vi "BMcalculate_v2_2.vi"() -> ()   [LabVIEW 2016]
uses:
  <vilib>/Analysis/coordinate.llb/2D Cartesian Coordinate Rotation (Array).vi
  <vilib>/Analysis/baseanly.llb/Mean (DBL).vi
  <vilib>/Utility/file.llb/Read From Spreadsheet File (string).vi
  <vilib>/Utility/file.llb/Write To Spreadsheet File (DBL).vi
  <vilib>/Analysis/NI_AALBase.lvlib
  <vilib>/Analysis/NI_AALPro.lvlib
panel:
  out "yBM (delete x/y,R2)":dbl[](array[numeric])
  out "xBM (delete x/y,R2)":dbl[](array[numeric])
  out "aoi count (delete x/y)":dbl[](array[numeric])
  out "y position (delete x/y)":dbl[][](array[numeric])
  out "yBM (delete x/y)":dbl[](array[numeric])
  out "xBM (delete x/y)":dbl[](array[numeric])
  out "x position (delete x/y)":dbl[][](array[numeric])
  out "aoi count":dbl[](array[numeric])
  out "aoi count repeat":dbl[](array[numeric])
  out "Tandem Yi position":dbl[](array[numeric])
  out "Tandem Xi position":dbl[](array[numeric])
  out "Time trace no hightlight":T1(graph)
  out "frame":i32
  out "BM":dbl[](array[numeric])
  out "sec":dbl[](array[numeric])
  out "y position (pixel) per aoi":dbl[](array[numeric])
  out "x position (pixel) per aoi":dbl[](array[numeric])
  out "final good yBM":dbl[](array[numeric])
  out "final good xBM":dbl[](array[numeric])
  out "final good aois (string)":string[](array[string])
  out "final good aoi (string)":string
  out "final good aois":dbl[](array[numeric])
  out "# of AOIs":dbl
  out "path out":path
  in  "(T=X , F=Y)":bool=TRUE
  in  "Filter window size":i32=100
  out "XYplot":path
  out "TimeTrace":path
  in  "Save Time-trace":bool
  in  "nm/pixel":dbl=72.5 format="%#_13g"
  in  "Folder path":path
  in  "?":bool
  in  "to":dbl=1.15 format="%#_13g"
  in  "x/y for all":dbl=0.85 format="%#_13g"
  out "filename":string
  in  "Filter mode":T2(ring)=enum."Median_slide window"
  in  "Save to vertical data ?":bool
  in  "?":enum32{"slide by slide", "delay"}(tab)=enum."delay"
  in  "?":bool
  in  "seconds to wait":u32
  in  "?":dbl=7.963 format="%#_13g"
  in  "?":dbl=48.61 format="%#_13g"
  in  "Save BM":bool
  in  "?":bool=TRUE
  in  "Save X-Y plot":bool
  in  "less than":dbl=0.2 format="%#_13g"
  in  "?":bool
  in  "?":bool
  in  "?":bool=TRUE
  out "# of frames":dbl
  in  "?":T3(tab)
  out "Filenames":string[](array[string])
  out "useful AOIs":i32[](array[numeric])
  out "# of AOI":i32[](array[numeric])
  out "% of useful AOIs":dbl
  out "tt # of AOIs":i32
  out "# of Frames":dbl[](array[numeric])
  out "tt # 0f useful AOIs":i32
  out "?":T4(graph)
  out "# of useful (each file)":i32
  out "X-Y plot":cluster{dbl[], dbl[]}(graph)
  out "Xstd":dbl
  out "ystd":dbl[](array[numeric])
  out "X":dbl format="%0.2f"
  out "Y":dbl format="%0.2f"
  out "?":T4(graph)
  out "tt # of useful AOIs":i32
  out "xstd":dbl[](array[numeric])
  out "all y position (pixel)":dbl[][](array[numeric])
  out "all x position (pixel)":dbl[][](array[numeric])
  out "Useful aoi number":string[][](array[string])
  in  "Tab Control":enum32{"Time trace"}(tab)
  out "Time trace":T1(graph)
  in  "Highlight":dbl=30.0
  in  "∮":dbl=30.0
  out "aoi":string
  in  "stop frame1":dbl
  in  "start frame1":dbl
  in  "start frame3":dbl
  in  "stop frame2":dbl
  in  "stop frame3":dbl
  in  "start frame2":dbl
  # "Critiria"
  # "∮"
  # "nm"
  # "for ssDNA strande exchange \n                    23.776∮6.613 nm"
  # "for D-loop  (90+4)\n                    48.61∮7.963 nm"
  # "for D-loop  (150+4)\n                    49.57∮8.56 nm"
  # "nm"
  # "Buffer wash"
  # "to"
  # "to"
  # "to"
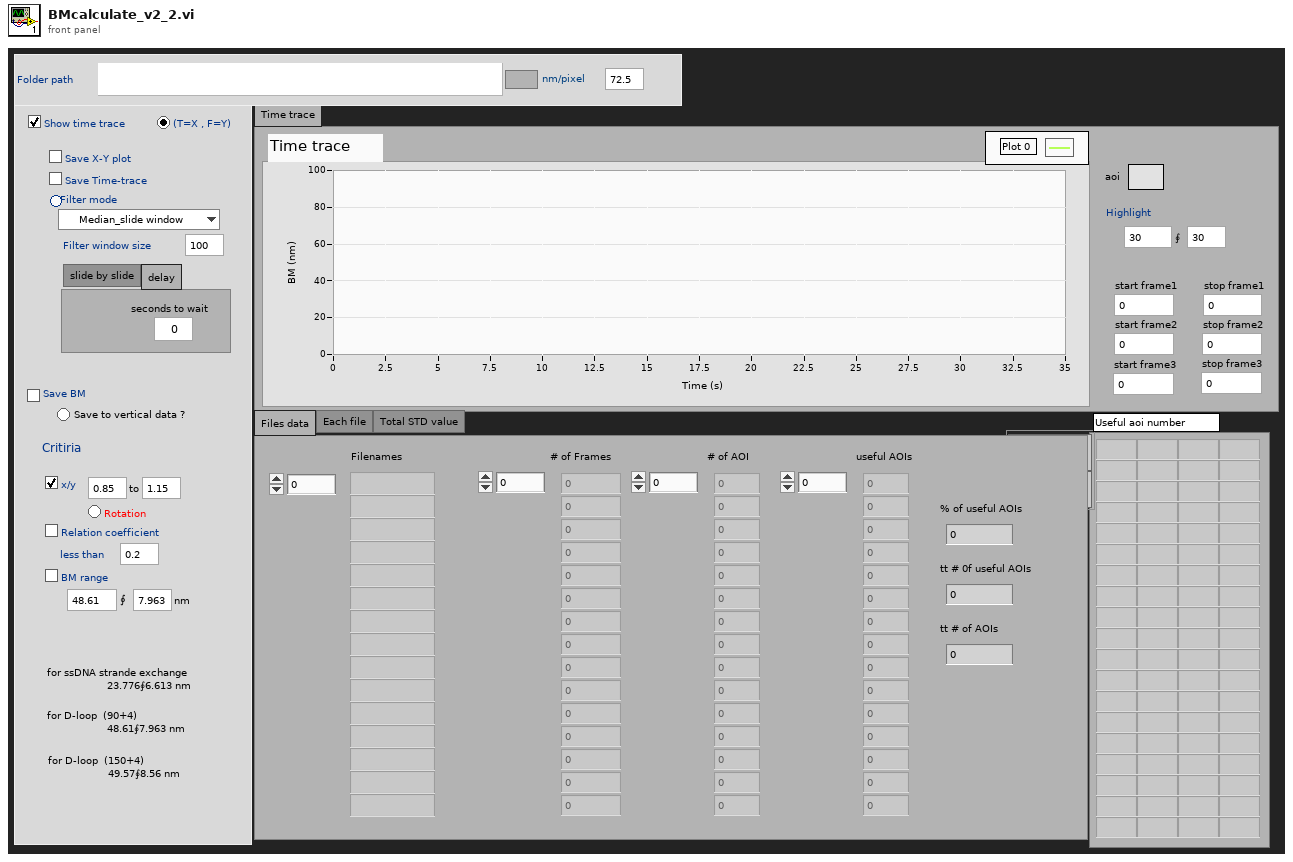
[diagram p1: front panel]
types:
  T1 = cluster{"Filtered X":dbl[], "Filtered X":dbl[]}[]
  T2 = enum16{"Median_fix window", "Average_fix window", "Median_slide window", "Average_slide window"}
  T3 = enum32{"Files data", "Each file", "Total STD value"}
  T4 = cluster{"X Values":dbl[], "Histogram: h(x)":i32[]}
  T5 = cluster{"y position (pixel) per aoi":dbl[], "x position (pixel) per aoi":dbl[]}
  T6 = cluster{"x position (pixel) per aoi":dbl[], "y position (pixel) per aoi":dbl[]}
  T7 = typedef "imagedata.ctl" = cluster{"image type":i32, "image depth":i32, "image":u8[], "mask":u8[], "colors":u32[], "Rectangle":cluster{"left":i16, "top":i16, "right":i16, "bottom":i16}}
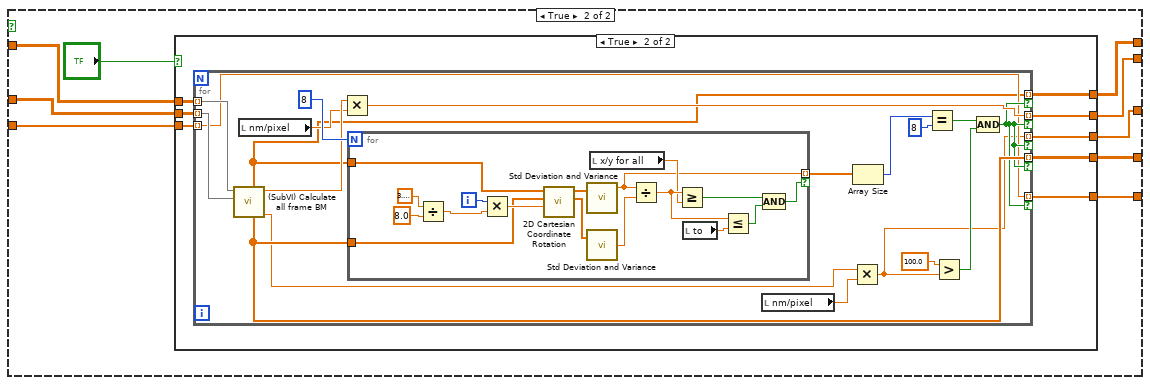
[diagram p3: hidden frame]
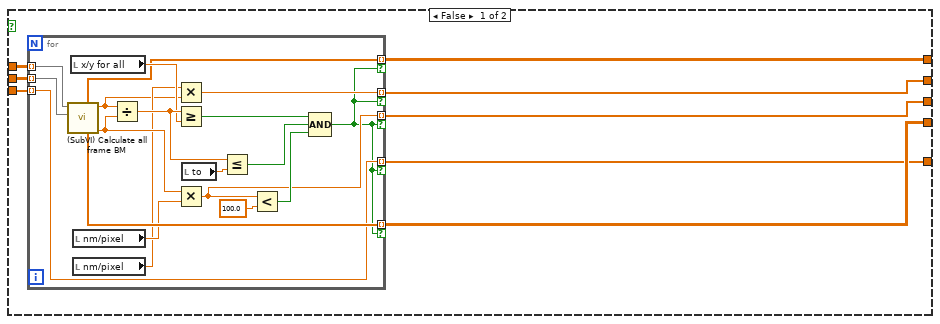
[diagram p4: hidden frame]
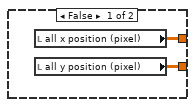
[diagram p7: hidden frame]
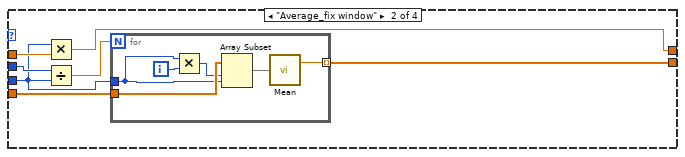
[diagram p9: hidden frame]
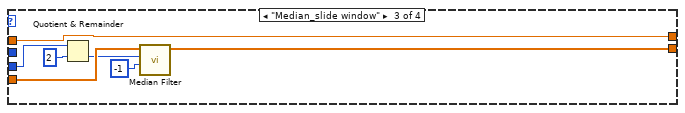
[diagram p10: hidden frame]
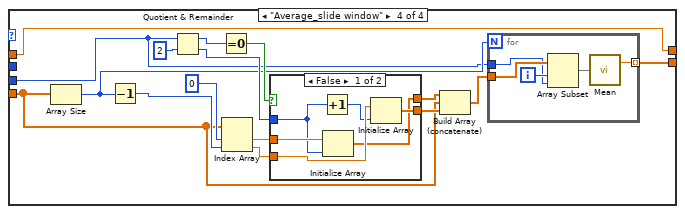
[diagram p11: hidden frame]
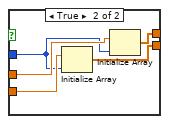
[diagram p12: hidden frame]
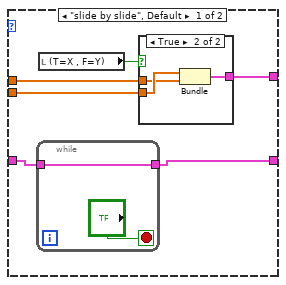
[diagram p13: hidden frame]
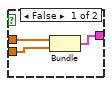
[diagram p14: hidden frame]
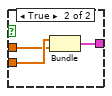
[diagram p15: hidden frame]
diagram:
  n1 = List Folder(path="Folder path", pattern="*.csv") -> (path out=→"path out":path, filenames=w3:string[])  [unwired: 2 in, 2 out]
  "Filenames" <- w3
  n2 = for {
    tunnel: w3 -> [w33] mode=indexing
    tunnel: [w32] -> w5 mode=concatenating
    tunnel: [w31] -> w21 mode=indexing
    tunnel: [w26] -> w20 mode=indexing
    tunnel: [w30] -> w13 mode=concatenating
    tunnel: [w25] -> w14 mode=indexing
    tunnel: [w27] -> w2 mode=indexing
    n3 = flat-sequence {
      tunnel: w33 -> [w45]
      tunnel: ["?"] -> w28
      tunnel: w28 -> [_]
      tunnel: [w193] -> w29
      tunnel: w29 -> [w221]
      tunnel: [w442] -> w30
      tunnel: [w443] -> w31
      tunnel: [w444] -> w32
      tunnel: [w441] -> w27
      tunnel: [w440] -> w26
      tunnel: [w439] -> w25
      frame #0 {
        n4 = local read "path out"() -> (w46:path)
        n5 = Build Path(base path=w46, name or relative path=w45) -> (appended path=w39:path)
        n6 = call "(SubVI) chnage name.vi"("replace \".csv\" to"="_TimeTrace" ("replace string (\"\")"), "Create path?"="Save Time-trace", "Folder path"=w39) -> ("created path"=→"TimeTrace":path)  [unwired: 8 in]
        n7 = call "(SubVI) chnage name.vi"("replace \".csv\" to"="_XYplot" ("replace string (\"\")"), "Create path?"="Save X-Y plot", "Folder path"=w39) -> ("created path"=→"XYplot":path)  [unwired: 8 in]
        n8 = call-poly <vilib>:"Read From Spreadsheet File.vi"("delimiter (\\t)"="," ("delimiter (\\t)"), "format (%s)"="%.4f" ("format (%.3f)"), "file path (dialog if empty)"=w39) -> ("all rows"=w63:string[][])  [unwired: 4 in, 4 out]
        n9 = Fract/Exp String To Number(string=w63) -> (number=w62:dbl[][])  [unwired: 3 in, 1 out]
        n10 = Index Array(array=w62, index (col) #1=8 ("disabled index (col)"), index (col) #2=9 ("index (col)"), index (col) #3=1 ("index (col)")) -> (element #1=w54:dbl[], element #2=w55:dbl[], element #3=w40:dbl[])  [unwired: 3 in]
        n11 = Delete From Array(array=w54, length=1, index=0) -> (array with subset deleted=→"Tandem Xi position":dbl[])  [unwired: 1 out]
        n12 = Delete From Array(array=w55, length=1, index=0) -> (array with subset deleted=→"Tandem Yi position":dbl[])  [unwired: 1 out]
        n13 = Delete From Array(array=w40, length=1, index=0) -> (array with subset deleted=w37:dbl[])  [unwired: 1 out]
        "aoi count repeat" <- w37
        n14 = Array Size(array=w37) -> (size(s)=w36:i32)
        n15 = Array Max & Min(array=w37) -> (max value=w35:dbl)  [unwired: 3 out]
        "# of AOIs" <- w35
        n16 = Divide(x=w36, y=w35) -> (x/y=→"# of frames":dbl)
        "filename" <- w45
      }
      frame #1 {
        n17 = local read "aoi count repeat"() -> (w68:dbl[])
        n18 = local read "# of AOIs"() -> (w75:dbl)
        n19 = local read "Tandem Xi position"() -> (w70:dbl[])
        n20 = local read "Tandem Yi position"() -> (w69:dbl[])
        n21 = local read "# of frames"() -> (w67:dbl)
        n22 = local read "# of frames"() -> (w66:dbl)
        n23 = local read "# of AOIs"() -> (w73:dbl)
        n24 = local read "# of AOIs"() -> (w74:dbl)
        n25 = Array Subset(array=w68, index=0, length=w75) -> (→"aoi count":dbl[])
        n26 = Reshape Array(w70, w67, w73) -> (w78:dbl[][])
        n27 = Reshape Array(w69, w66, w74) -> (w79:dbl[][])
        n28 = Transpose 2D Array(2D array=w78) -> (transposed array=→"all x position (pixel)":dbl[][])
        n29 = Transpose 2D Array(2D array=w79) -> (transposed array=→"all y position (pixel)":dbl[][])
      }
      frame #2 {
        n30 = local read "all x position (pixel)"() -> (w85:dbl[][])
        n31 = local read "all y position (pixel)"() -> (w84:dbl[][])
        n32 = local read "aoi count"() -> (w83:dbl[])
        n33 = case shown="False" "?" {
          tunnel: [w96 w114] -> w88
          tunnel: [w95 w113] -> w81
          tunnel: w85 -> [w99 w112]
          tunnel: w84 -> [w98 w111]
          tunnel: [w92 w107] -> w87
          tunnel: [w89 w106] -> w82
          tunnel: w83 -> [w97 w109]
          tunnel: [w97 w108] -> w80
          frame False {
            n34 = for {
              tunnel: w99 -> [w105] mode=indexing
              tunnel: w98 -> [w104] mode=indexing
              tunnel: [w103] -> w94 mode=indexing
              tunnel: [w102] -> w90 mode=indexing
              tunnel: [w101] -> w96 mode=indexing
              tunnel: [w100] -> w95 mode=indexing
              n35 = call "(SubVI) Calculate all frame BM.vi"("y position (pixel)"=w104, "x position (pixel)"=w105) -> ("y standard deviation"=w102:dbl, "x standard deviation"=w103:dbl, "y position (delete y fit error)"=w100:dbl[], "x position (delete x fit error)"=w101:dbl[])  [unwired: 6 in]
            }
            n36 = local read "nm/pixel"() -> (w93:dbl)
            n37 = local read "nm/pixel"() -> (w91:dbl)
            n38 = Multiply(x=w94, y=w93) -> (x*y=w92:dbl[])
            n39 = Multiply(x=w91, y=w90) -> (x*y=w89:dbl[])
          }
          frame True {
            n40 = case shown="True" "?" {
              tunnel: w111 -> [w121 w149]
              tunnel: w112 -> [w122 w148]
              tunnel: [w120 w144] -> w114
              tunnel: [w119 w143] -> w113
              tunnel: [w118 w147] -> w106
              tunnel: [w117 w146] -> w107
              tunnel: w109 -> [w116 w145]
              tunnel: [w115 w142] -> w108
              frame False {
                n41 = for {
                  tunnel: w122 -> [w132] mode=indexing
                  tunnel: w121 -> [w131] mode=indexing
                  tunnel: [w129] -> w120 mode=indexing if=w123
                  tunnel: [w128] -> w119 mode=indexing if=w123
                  tunnel: [w133] -> w118 mode=indexing if=w123
                  tunnel: [w136] -> w117 mode=indexing if=w123
                  tunnel: w116 -> [w127] mode=indexing
                  tunnel: [w127] -> w115 mode=indexing if=w123
                  n42 = call "(SubVI) Calculate all frame BM.vi"("y position (pixel)"=w131, "x position (pixel)"=w132) -> ("y standard deviation"=w130:dbl, "x standard deviation"=w124:dbl, "y position (delete y fit error)"=w128:dbl[], "x position (delete x fit error)"=w129:dbl[])  [unwired: 6 in]
                  n43 = local read "x/y for all"() -> (w140:dbl)
                  n44 = local read "nm/pixel"() -> (w126:dbl)
                  n45 = local read "nm/pixel"() -> (w125:dbl)
                  n46 = Divide(x=w124, y=w130) -> (x/y=w141:dbl)
                  n47 = Multiply(x=w125, y=w124) -> (x*y=w136:dbl)
                  n48 = Greater Or Equal?(x=w141, y=w140) -> (x >= y?=w138:bool)
                  n49 = Multiply(x=w130, y=w126) -> (x*y=w133:dbl)
                  n50 = local read "to"() -> (w139:dbl)
                  n51 = Less Or Equal?(x=w141, y=w139) -> (x <= y?=w137:bool)
                  n52 = Less?(x=w133, y=100.0) -> (x < y?=w134:bool)
                  n53 = Compound Arithmetic op=AND(w138, w137, w134) -> (w123:bool)
                }
              }
              frame True {
                n54 = for {
                  tunnel: w148 -> [w168] mode=indexing
                  tunnel: w149 -> [w167] mode=indexing
                  tunnel: [w151] -> w147 mode=indexing if=w157
                  tunnel: [w152] -> w144 mode=indexing if=w157
                  tunnel: [w162] -> w143 mode=indexing if=w157
                  tunnel: [w160] -> w146 mode=indexing if=w157
                  tunnel: [w156] -> w142 mode=indexing if=w157
                  tunnel: w145 -> [w156] mode=indexing
                  n55 = call "(SubVI) Calculate all frame BM.vi"("y position (pixel)"=w167, "x position (pixel)"=w168) -> ("y standard deviation"=w154:dbl, "x standard deviation"=w161:dbl, "y position (delete y fit error)"=w162:dbl[], "x position (delete x fit error)"=w152:dbl[])  [unwired: 6 in]
                  n56 = local read "nm/pixel"() -> (w153:dbl)
                  n57 = Multiply(x=w161, y=w153) -> (x*y=w160:dbl)
                  n58 = for {
                    N: 8 -> [_]
                    tunnel: w162 -> [w170]
                    tunnel: w152 -> [w171]
                    tunnel: [w169] -> w163 mode=indexing if=w174
                    i -> [w181]
                    n59 = Divide(x=3.141592653589793, y=8.0) -> (x/y=w184:dbl)
                    n60 = Multiply(x=w181, y=w184) -> (x*y=w182:dbl)
                    n61 = call-poly <vilib>:"2D Cartesian Coordinate Rotation.vi"("theta"=w182, "Y"=w170, "X"=w171) -> ("Y Out"=w175:dbl[], "X Out"=w176:dbl[])  [unwired: 6 in, 1 out]
                    n62 = call <vilib>:"Std Deviation and Variance.vi"("X"=w176) -> ("mean"=w169:dbl)  [unwired: 1 in, 2 out]
                    n63 = call <vilib>:"Std Deviation and Variance.vi"("X"=w175) -> ("standard deviation"=w180:dbl)  [unwired: 1 in, 2 out]
                    n64 = local read "x/y for all"() -> (w173:dbl)
                    n65 = Divide(x=w169, y=w180) -> (x/y=w179:dbl)
                    n66 = Greater Or Equal?(x=w179, y=w173) -> (x >= y?=w178:bool)
                    n67 = local read "to"() -> (w172:dbl)
                    n68 = Less Or Equal?(x=w179, y=w172) -> (x <= y?=w177:bool)
                    n69 = Compound Arithmetic op=AND(w178, w177) -> (w174:bool)
                  }
                  n70 = local read "nm/pixel"() -> (w155:dbl)
                  n71 = Multiply(x=w154, y=w155) -> (x*y=w151:dbl)
                  n72 = Array Size(array=w163) -> (size(s)=w165:i32)
                  n73 = Equal?(x=w165, y=8) -> (x = y?=w158:bool)
                  n74 = Greater?(x=100.0 ("y"), y=w151) -> (0:w159:bool)
                  n75 = Compound Arithmetic op=AND(w158, w159) -> (w157:bool)
                }
              }
            }
          }
        }
        "x position (delete x/y)" <- w88
        "xBM (delete x/y)" <- w87
        "yBM (delete x/y)" <- w82
        "y position (delete x/y)" <- w81
        "aoi count (delete x/y)" <- w80
      }
      frame #3 {
        n76 = local read "x position (delete x/y)"() -> (w192:dbl[][])
        n77 = local read "y position (delete x/y)"() -> (w189:dbl[][])
        n78 = local read "aoi count (delete x/y)"() -> (w188:dbl[])
        n79 = local read "yBM (delete x/y)"() -> (w190:dbl[])
        n80 = local read "xBM (delete x/y)"() -> (w191:dbl[])
        n81 = case shown="True" "?" {
          tunnel: w192 -> [_ w205]
          tunnel: w189 -> [_ w204]
          tunnel: w191 -> [w197 w203]
          tunnel: w190 -> [w196 w201]
          tunnel: [w197 w202] -> w187
          tunnel: [w196 w200] -> w186
          tunnel: w188 -> [w195 w199]
          tunnel: [w195 w198] -> w193
          frame False {
          }
          frame True {
            n82 = for {
              tunnel: w205 -> [w211] mode=indexing
              tunnel: w204 -> [w210] mode=indexing
              tunnel: [w206] -> w202 mode=indexing if=w208
              tunnel: w203 -> [w206] mode=indexing
              tunnel: w201 -> [w207] mode=indexing
              tunnel: [w207] -> w200 mode=indexing if=w208
              tunnel: [w209] -> w198 mode=indexing if=w208
              tunnel: w199 -> [w209] mode=indexing
              n83 = call "(SubVI) Calculate xy correlation.vi"("y position (delete y fit error)"=w210, "x position (delete x fit error)"=w211) -> ("Numeric"=w212:dbl)  [unwired: 9 in]
              n84 = Less Or Equal?(x=w212, y="less than") -> (x <= y?=w208:bool)
            }
          }
        }
        "xBM (delete x/y,R2)" <- w187
        "yBM (delete x/y,R2)" <- w186
      }
      frame #4 {
        n85 = local read "xBM (delete x/y,R2)"() -> (w215:dbl[])
        n86 = local read "xBM (delete x/y,R2)"() -> (w214:dbl[])
        n87 = case shown="True" "?" {
          tunnel: w215 -> [w225 w231]
          tunnel: [w225 w230] -> w216
          tunnel: w214 -> [w224 w229]
          tunnel: [w224 w228] -> w219
          tunnel: w221 -> [w223 w227]
          tunnel: [w223 w226] -> w220
          frame False {
          }
          frame True {
            n88 = for {
              tunnel: [w232] -> w230 mode=indexing if=w238
              tunnel: w231 -> [w232] mode=indexing
              tunnel: w229 -> [w237] mode=indexing
              tunnel: [w237] -> w228 mode=indexing if=w238
              tunnel: [w239] -> w226 mode=indexing if=w238
              tunnel: w227 -> [w239] mode=indexing
              n89 = Subtract(x="?", y="?") -> (x-y=w234:dbl)
              n90 = Add(x="?", y="?") -> (x+y=w233:dbl)
              n91 = Greater Or Equal?(x=w232, y=w234) -> (x >= y?=w241:bool)
              n92 = Less Or Equal?(x=w232, y=w233) -> (x <= y?=w240:bool)
              n93 = Compound Arithmetic op=AND(w241, w240) -> (w238:bool)
            }
          }
        }
        "final good aois" <- w220
        "final good xBM" <- w216
        "final good yBM" <- w219
        n94 = call <vilib>:"Histogram.vi"("X"=w216) -> ("Histogram Graph"=→"?":T4)  [unwired: 7 in, 3 out]
        n95 = Array Size(array=w216) -> (size(s)=→"# of useful (each file)":i32)
      }
      frame #5 {
        n96 = case shown="True" "(T=X , F=Y)" {
          tunnel: [w249 w251] -> w245
          tunnel: [w248 w250] -> w244
          frame False {
            n97 = local read "all x position (pixel)"() -> (w248:dbl[][])
            n98 = local read "all y position (pixel)"() -> (w249:dbl[][])
          }
          frame True {
            n99 = local read "all y position (pixel)"() -> (w250:dbl[][])
            n100 = local read "all x position (pixel)"() -> (w251:dbl[][])
          }
        }
        n101 = local read "final good aois"() -> (w243:dbl[])
        n102 = local read "final good xBM"() -> (w242:dbl[])
        n103 = Number To Decimal String(number=w243) -> (decimal integer string=w247:string[])  [unwired: 1 in]
        "final good aois (string)" <- w247
        n104 = for {
          tunnel: w245 -> [w253] mode=indexing
          tunnel: w244 -> [w252] mode=indexing
          tunnel: w247 -> [w254] mode=indexing
          tunnel: w242 -> [w255] mode=indexing
          n105 = case shown="True" "?" {
            frame False {
            }
            frame True {
              n106 = flat-sequence {
                tunnel: "Tab Control" -> [_]
                frame #0 {
                  n107 = local read "x position (pixel) per aoi"() -> (w262:dbl[])
                  n108 = local read "nm/pixel"() -> (w259:dbl)
                  n109 = call "(SubVI) Calculate window frame BM.vi"("nm/pixel"=w259, "all x position (pixel)"=w262) -> ("BM"=→"BM":dbl[], "sec"=→"sec":dbl[], "frame"=→"frame":i32)  [unwired: 3 in]
                }
                frame #1 {
                  n110 = local read "frame"() -> (w267:i32)
                  n111 = local read "BM"() -> (w265:dbl[])
                  n112 = Reciprocal(x=30.0) -> (1/x=w276:dbl)
                  n113 = case shown="\"Median_fix window\", Default" "Filter mode" {
                    tunnel: [w292 w303 w318 w335] -> w274
                    tunnel: w265 -> [w293 w304 w319 w324]
                    tunnel: w267 -> [w291 w306 _ _]
                    tunnel: "Filter window size" -> [w287 w300 w315 w321]
                    tunnel: w276 -> [w289 w302 w317 w320]
                    tunnel: [w288 w301 w317 w320] -> w275
                    frame "Median_fix window", Default {
                      n114 = Multiply(x=w289, y=w287) -> (x*y=w288:dbl)
                      n115 = Divide(x=w291, y=w287) -> (x/y=w290:dbl)
                      n116 = for {
                        N: w290 -> [_]
                        tunnel: w293 -> [w299]
                        tunnel: [w297] -> w292 mode=indexing
                        tunnel: w287 -> [w294]
                        tunnel: w289 -> [_]
                        i -> [w296]
                        n117 = Multiply(x=w294, y=w296) -> (x*y=w295:i32)
                        n118 = Array Subset(array=w299, index=w295, length=w294) -> (w298:dbl[])
                        n119 = call <vilib>:"Median.vi"("X"=w298) -> ("median"=w297:dbl)  [unwired: 1 out]
                      }
                    }
                    frame "Average_fix window" {
                      n120 = Multiply(x=w300, y=w302) -> (x*y=w301:dbl)
                      n121 = Divide(x=w306, y=w300) -> (x/y=w305:dbl)
                      n122 = for {
                        N: w305 -> [_]
                        tunnel: w304 -> [w312]
                        tunnel: [w310] -> w303 mode=indexing
                        tunnel: w300 -> [w308]
                        i -> [w309]
                        n123 = Multiply(x=w308, y=w309) -> (x*y=w307:i32)
                        n124 = Array Subset(array=w312, index=w307, length=w308) -> (w311:dbl[])
                        n125 = call-poly <vilib>:"Mean.vi"("X"=w311) -> ("mean"=w310:dbl)  [unwired: 1 out]
                      }
                    }
                    frame "Median_slide window" {
                      n126 = Quotient & Remainder(x=w315, y=2) -> (floor(x/y)=w313:i32)  [unwired: 1 out]
                      n127 = call <vilib>:"Median Filter.vi"("right rank"=-1, "left rank"=w313, "X"=w319) -> ("Filtered X"=w318:dbl[])  [unwired: 7 in, 1 out]
                    }
                    frame "Average_slide window" {
                      n128 = Array Size(array=w324) -> (size(s)=w322:i32)
                      n129 = Decrement(x=w322) -> (x-1=w328:i32)
                      n130 = Quotient & Remainder(x=w321, y=2) -> (x-y*floor(x/y)=w331:i32, floor(x/y)=w329:i32)
                      n131 = Equal To 0?(x=w331) -> (x = 0?=w330:bool)
                      n132 = Index Array(array=w324, index #1=0 ("index"), index #2=w328) -> (element #1=w333:dbl, element #2=w327:dbl)
                      n133 = case shown="False" w330 {
                        tunnel: w333 -> [w341 w346]
                        tunnel: w329 -> [w338 w344]
                        tunnel: w327 -> [w340 w345]
                        tunnel: [w336 w343] -> w326
                        tunnel: [w337 w342] -> w325
                        frame False {
                          n134 = Increment(x=w338) -> (x+1=w339:i32)
                          n135 = Initialize Array(w341, w338) -> (w336:dbl[])
                          n136 = Initialize Array(w340, w339) -> (w337:dbl[])
                        }
                        frame True {
                          n137 = Initialize Array(w345, w344) -> (w342:dbl[])
                          n138 = Initialize Array(w346, w344) -> (w343:dbl[])
                        }
                      }
                      n139 = Build Array (concatenate)(w326, w324, w325) -> (w323:dbl[])
                      n140 = for {
                        N: w322 -> [_]
                        tunnel: w323 -> [w351]
                        tunnel: [w349] -> w335 mode=indexing
                        tunnel: w321 -> [w347]
                        i -> [w348]
                        n141 = Array Subset(array=w351, index=w348, length=w347) -> (w350:dbl[])
                        n142 = call-poly <vilib>:"Mean.vi"("X"=w350) -> ("mean"=w349:dbl)  [unwired: 1 out]
                      }
                    }
                  }
                  n143 = call "(SubVI) Calculate time.vi"("dt"=w275, "BM"=w274) -> ("Time (s)"=w273:dbl[])  [unwired: 3 in]
                  n144 = for {
                    tunnel: w274 -> [w284] mode=indexing
                    tunnel: [w284] -> w271 mode=indexing if=w285
                    tunnel: w273 -> [w286] mode=indexing
                    tunnel: [w286] -> w272 mode=indexing if=w285
                    n145 = Not Equal To 0?(x=w284) -> (x != 0?=w285:bool)
                  }
                  n146 = local read "sec"() -> (w268:dbl[])
                  n147 = local read "BM"() -> (w266:dbl[])
                  n148 = local read "y position (pixel) per aoi"() -> (w269:dbl[])
                  n149 = local read "x position (pixel) per aoi"() -> (w270:dbl[])
                  n150 = Bundle("sec"=w268, "BM"=w266) -> (w280:cluster{"sec":dbl[], "BM":dbl[]})  [unwired: 1 in]
                  n151 = Bundle(w272, w271) -> (w283:cluster{dbl[], dbl[]})  [unwired: 1 in]
                  n152 = Build Array(w283, w280) -> (w263:cluster{"sec":dbl[], "BM":dbl[]}[])
                  n153 = case shown="\"delay\"" "?" {
                    tunnel: w263 -> [w357 w373]
                    tunnel: [w356 w373] -> w264
                    tunnel: w270 -> [w355 w369]
                    tunnel: w269 -> [w354 w368]
                    tunnel: [w353 w367] -> w279
                    frame "slide by slide", Default {
                      n154 = while {
                        tunnel: w357 -> [w364]
                        tunnel: [w364] -> w356
                        stop <- "?" stop-if-true
                      }
                      n155 = local read "(T=X , F=Y)"() -> (w352:bool)
                      n156 = case shown="True" w352 {
                        tunnel: w355 -> [w360 w363]
                        tunnel: w354 -> [w359 w362]
                        tunnel: [w358 w361] -> w353
                        frame False {
                          n157 = Bundle("y position (pixel) per aoi"=w359, "x position (pixel) per aoi"=w360) -> (w358:T5)  [unwired: 1 in]
                        }
                        frame True {
                          n158 = Bundle("x position (pixel) per aoi"=w363, "y position (pixel) per aoi"=w362) -> (w361:T6)  [unwired: 1 in]
                        }
                      }
                    }
                    frame "delay" {
                      n159 = local read "(T=X , F=Y)"() -> (w366:bool)
                      n160 = case shown="False" w366 {
                        tunnel: w369 -> [w376 w379]
                        tunnel: w368 -> [w375 w378]
                        tunnel: [w374 w377] -> w367
                        frame False {
                          n161 = Bundle("y position (pixel) per aoi"=w375, "x position (pixel) per aoi"=w376) -> (w374:T5)  [unwired: 1 in]
                        }
                        frame True {
                          n162 = Bundle("x position (pixel) per aoi"=w379, "y position (pixel) per aoi"=w378) -> (w377:T6)  [unwired: 1 in]
                        }
                      }
                      n163 = Multiply(x="seconds to wait", y=u32 1000) -> (x*y=w371:u32)
                      n164 = Wait (ms)(milliseconds to wait=w371) -> ()  [unwired: 1 out]
                    }
                  }
                  "X-Y plot" <- w279
                  "Time trace no hightlight" <- w264
                }
                frame #2 {
                  (unwired) 300
                  n165 = local read "sec"() -> (w414:dbl[])
                  n166 = local read "sec"() -> (w415:dbl[])
                  n167 = Subtract(x="Highlight", y="∮") -> (x-y=w386:dbl)
                  n168 = Add(x="Highlight", y="∮") -> (x+y=w387:dbl)
                  n169 = call "(SubVI) frame to time(s).vi"("Numeric in"="start frame2") -> ("Numeric out"=w408:dbl)  [unwired: 10 in]
                  n170 = call "(SubVI) frame to time(s).vi"("Numeric in"="stop frame2") -> ("Numeric out"=w409:dbl)  [unwired: 10 in]
                  n171 = call "(SubVI) frame to time(s).vi"("Numeric in"="start frame3") -> ("Numeric out"=w412:dbl)  [unwired: 10 in]
                  n172 = call "(SubVI) frame to time(s).vi"("Numeric in"="stop frame3") -> ("Numeric out"=w413:dbl)  [unwired: 10 in]
                  n173 = call "(SubVI) frame to time(s).vi"("Numeric in"="start frame1") -> ("Numeric out"=w402:dbl)  [unwired: 10 in]
                  n174 = call "(SubVI) frame to time(s).vi"("Numeric in"="stop frame1") -> ("Numeric out"=w405:dbl)  [unwired: 10 in]
                  n175 = Array Size(array=w414) -> (size(s)=w392:i32)
                  n176 = local read "Time trace no hightlight"() -> (w416:T1)
                  n177 = Initialize Array(w408, w392) -> (w394:dbl[])
                  n178 = Initialize Array(w409, w392) -> (w395:dbl[])
                  n179 = Initialize Array(w412, w392) -> (w396:dbl[])
                  n180 = Initialize Array(w413, w392) -> (w397:dbl[])
                  n181 = Initialize Array(w402, w392) -> (w388:dbl[])
                  n182 = Initialize Array(w405, w392) -> (w389:dbl[])
                  n183 = Initialize Array(w386, w392) -> (w381:dbl[])
                  n184 = Initialize Array(w387, w392) -> (w382:dbl[])
                  n185 = Bundle(w394, "sec"=w414) -> (w398:cluster{dbl[], "sec":dbl[]})  [unwired: 1 in]
                  n186 = Bundle(w395, "sec"=w414) -> (w399:cluster{dbl[], "sec":dbl[]})  [unwired: 1 in]
                  n187 = Bundle(w396, "sec"=w414) -> (w400:cluster{dbl[], "sec":dbl[]})  [unwired: 1 in]
                  n188 = Bundle(w397, "sec"=w415) -> (w401:cluster{dbl[], "sec":dbl[]})  [unwired: 1 in]
                  n189 = Bundle(w388, "sec"=w414) -> (w390:cluster{dbl[], "sec":dbl[]})  [unwired: 1 in]
                  n190 = Bundle(w389, "sec"=w414) -> (w391:cluster{dbl[], "sec":dbl[]})  [unwired: 1 in]
                  n191 = Bundle("sec"=w414, w381) -> (w380:cluster{"sec":dbl[], dbl[]})  [unwired: 1 in]
                  n192 = Bundle("sec"=w414, w382) -> (w383:cluster{"sec":dbl[], dbl[]})  [unwired: 1 in]
                  n193 = Build Array (concatenate)(w398, w399, w400, w401, w390, w391, w416, w380, w383) -> (→"Time trace":cluster{"sec":dbl[], "Filtered X":dbl[]}[])
                }
                frame #3 {
                  n194 = local read "final good aoi (string)"() -> (w417:string)
                  n195 = local read "final good aoi (string)"() -> (w418:string)
                  n196 = local read "Save Time-trace"() -> (w423:bool)
                  n197 = local read "Save X-Y plot"() -> (w421:bool)
                  n198 = local read "TimeTrace"() -> (w422:path)
                  n199 = local read "XYplot"() -> (w420:path)
                  n200 = case shown="True" w421 {
                    tunnel: w417 -> [_ w430]
                    tunnel: w420 -> [_ w427]
                    frame False {
                    }
                    frame True {
                      n201 = Concatenate Strings("aoi" ("string"), w430, ".jpeg" ("string")) -> (w428:string)
                      n202 = invoke on="X-Y plot" class="XYGraph (strict)" method="Get Image"() -> ("image data"=w425:T7)  [unwired: 6 in, 5 out]
                      n203 = Build Path(base path=w427, name or relative path=w428) -> (appended path=w426:path)
                      n204 = call <vilib>:"Write JPEG File.vi"("image data"=w425, "path to JPEG file"=w426) -> ()  [unwired: 8 in, 2 out]
                    }
                  }
                  n205 = case shown="True" w423 {
                    tunnel: w418 -> [w431 w433]
                    tunnel: w422 -> [_ w436]
                    tunnel: [w431 w433] -> w419
                    frame False {
                    }
                    frame True {
                      n206 = Concatenate Strings("aoi" ("string"), w433, ".jpeg" ("string")) -> (w437:string)
                      n207 = invoke on="Time trace" class="XYGraph (strict)" method="Get Image"() -> ("image data"=w432:T7)  [unwired: 6 in, 5 out]
                      n208 = Build Path(base path=w436, name or relative path=w437) -> (appended path=w435:path)
                      n209 = call <vilib>:"Write JPEG File.vi"("image data"=w432, "path to JPEG file"=w435) -> ()  [unwired: 8 in, 2 out]
                    }
                  }
                  "aoi" <- w419
                }
              }
            }
          }
          "Xstd" <- w255
          "final good aoi (string)" <- w254
          "x position (pixel) per aoi" <- w253
          "y position (pixel) per aoi" <- w252
        }
      }
      frame #6 {
        n210 = local read "final good aois (string)"() -> (w441:string[])
        n211 = local read "# of useful (each file)"() -> (w443:i32)
        n212 = local read "final good yBM"() -> (w442:dbl[])
        n213 = local read "final good xBM"() -> (w444:dbl[])
        n214 = local read "# of frames"() -> (w439:dbl)
        n215 = local read "# of AOIs"() -> (w440:dbl)
      }
    }
  }
  "useful AOIs" <- w21
  "# of AOI" <- w20
  "ystd" <- w13
  "# of Frames" <- w14
  "xstd" <- w5
  n216 = Add Array Elements(numeric array=w21) -> (sum=w19:i32)
  n217 = Add Array Elements(numeric array=w20) -> (sum=w18:dbl)
  "tt # of AOIs" <- w18
  n218 = call-poly <vilib>:"Mean.vi"("X"=w13) -> ("mean"=→"Y":dbl)  [unwired: 1 out]
  n219 = Transpose 2D Array(2D array=w2) -> (transposed array=→"Useful aoi number":string[][])
  n220 = Array Size(array=w5) -> (size(s)=w10:i32)
  "tt # 0f useful AOIs" <- w10
  "tt # of useful AOIs" <- w10
  n221 = call-poly <vilib>:"Mean.vi"("X"=w5) -> ("mean"=→"X":dbl)  [unwired: 1 out]
  n222 = call <vilib>:"Histogram.vi"("X"=w5) -> ("Histogram Graph"=→"?":T4)  [unwired: 7 in, 3 out]
  n223 = Divide(x=w19, y=w18) -> (x/y=w17:dbl)
  n224 = Number To Decimal String(number=w10) -> (decimal integer string=w9:string)  [unwired: 1 in]
  n225 = Concatenate Strings("\\" ("string"), w9) -> (w4:string)
  n226 = Multiply(x=w17, y=100.0) -> (x*y=→"% of useful AOIs":dbl)
  n227 = case shown="True" "Save BM" {
    tunnel: w5 -> [_ w452]
    tunnel: w4 -> [_ w446]
    frame False {
    }
    frame True {
      n228 = local read "Folder path"() -> (w451:path)
      n229 = Path To String(path=w451) -> (string=w450:string)
      n230 = Concatenate Strings(w450, w446, ".txt" ("string")) -> (w449:string)
      n231 = String To Path(string=w449) -> (path=w448:path)
      n232 = call-poly <vilib>:"Write To Spreadsheet File.vi"("transpose? (no:F)"="Save to vertical data ?", "1D data"=w452, "file path (dialog if empty)"=w448) -> ()  [unwired: 5 in, 1 out]
    }
  }
